vi "Test Target Angle Correction.vi"() -> ()   [LabVIEW 2011]
panel:
  in  "Target Width":dbl
  in  "Recursive Iterations":dbl
  out "Angle Target Compensated":dbl
  out "Angle To Target Compensated":dbl(knob) scale=-90.0..90.0
  out "Angle Target":dbl
  out "Angle To Target":dbl(knob) scale=-90.0..90.0
  in  "Depth Lead":dbl
  out "Compound Backboard Depth":dbl
  in  "Right Target Depth":dbl
  in  "Left target depth":dbl
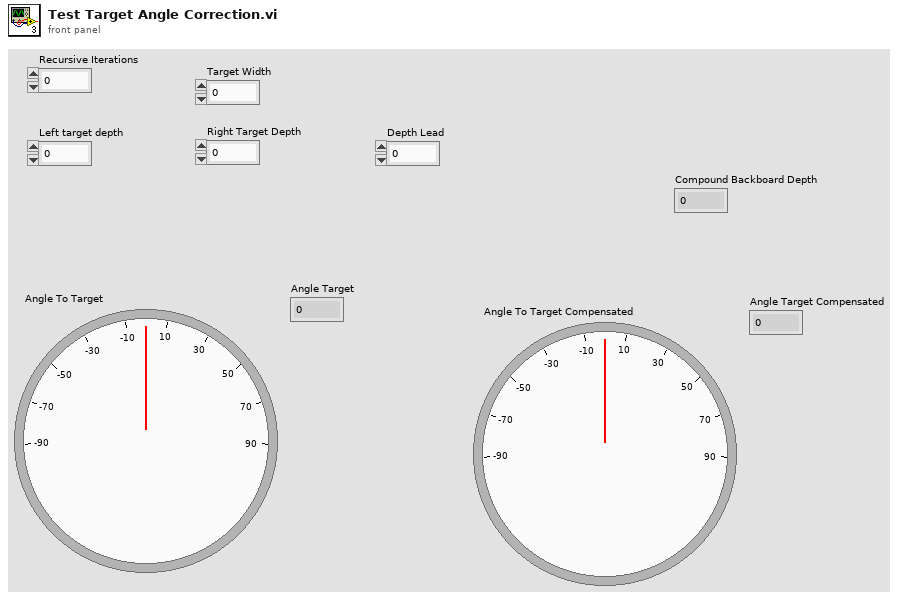
[diagram p1: front panel]
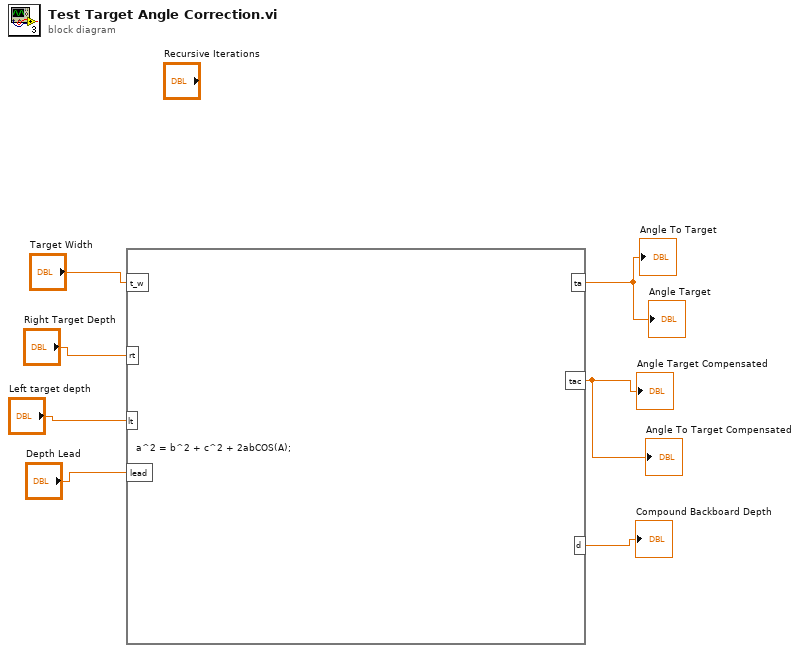
[diagram p0: block diagram]
diagram:
  n1 = formula code="a^2 = b^2 + c^2 + 2abCOS(A);"("t_w"="Target Width", "rt"="Right Target Depth", "lt"="Left target depth", "lead"="Depth Lead") -> ("ta"=→"Angle To Target" →"Angle Target":dbl, "tac"=→"Angle To Target Compensated" →"Angle Target Compensated":dbl, "d"=→"Compound Backboard Depth":dbl)
